vi "Capture System Configuration.vi"() -> ()   [LabVIEW 2024]
uses:
  <vilib>/Plug-In SDKs/Clients/Metadata/Test Station.ctl
  <vilib>/Plug-In SDKs/Clients/Metadata/Extension.ctl
  <vilib>/Plug-In SDKs/Clients/Metadata/Hardware Item.ctl
  <vilib>/Plug-In SDKs/Clients/Metadata/Software Item.ctl
  <vilib>/Plug-In SDKs/Clients/Metadata/Operator.ctl
  <vilib>/Plug-In SDKs/Clients/Data Store V1/Data Store Client.lvlibp/API/Data Store V1/Test Result.ctl
  <vilib>/Plug-In SDKs/Clients/Metadata/Outcome.ctl
  <vilib>/Plug-In SDKs/Clients/Metadata Store V1/Metadata Store Client.lvlibp/API/Metadata Store V1/Create Hardware Item.vi
  <vilib>/nisyscfg/Get Installed Components.vi
  <vilib>/Plug-In SDKs/Clients/Metadata Store V1/Metadata Store Client.lvlibp/API/Metadata Store V1/Create Software Item.vi
  <vilib>/Plug-In SDKs/Clients/Metadata Store V1/Metadata Store Client.lvlibp/API/Metadata Store V1/Create Test Station.vi
  <vilib>/Plug-In SDKs/Clients/Metadata Store V1/Metadata Store Client.lvlibp/API/Metadata Store V1/Create Operator.vi
  <vilib>/nisyscfg/nisyscfg.lvlib
  <resource>/objmgr/nisysapi.rc
  <vilib>/Plug-In SDKs/Clients/Metadata Store V1/Metadata Store Client.lvlibp
  <vilib>/Plug-In SDKs/Clients/Metadata/NI Metadata Types.lvlib
  <vilib>/Plug-In SDKs/Clients/Data Store V1/Data Store Client.lvlibp
panel:
  out "found operator":T1
  out "found software items":T3[](array[typedef])
  out "found hardware items":T4[](array[typedef])
  out "found test station":T5
  out "queried data":waveform(dbl)(graph)
  out "error out":errorcluster
  # "Capture System Configuration\n\nThis example uses System API to query information about the current system and create metadata items based on that information. A waveform measurement is published, then the data and metadata are read back from the published measurement."
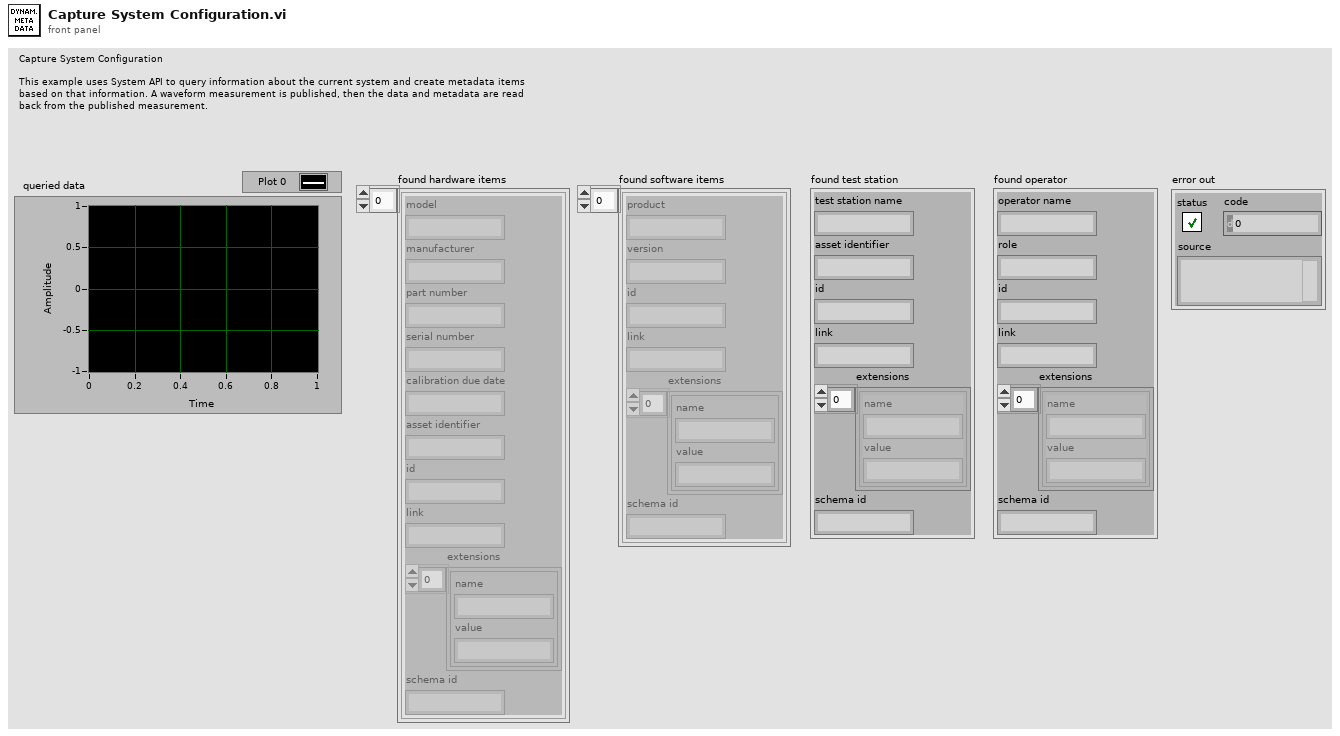
[diagram p1: front panel]
types:
  T1 = typedef "NI Metadata Types.lvlib/Operator.ctl" = cluster{"operator name":string, "role":string, "id":string, "link":string, "extensions":T2[], "schema id":string}
  T2 = typedef "NI Metadata Types.lvlib/Extension.ctl" = cluster{"name":string, "value":string}
  T3 = typedef "NI Metadata Types.lvlib/Software Item.ctl" = cluster{"product":string, "version":string, "id":string, "link":string, "extensions":T2[], "schema id":string}
  T4 = typedef "NI Metadata Types.lvlib/Hardware Item.ctl" = cluster{"model":string, "manufacturer":string, "part number":string, "serial number":string, "calibration due date":string, "asset identifier":string, "id":string, "link":string, "extensions":T2[], "schema id":string}
  T5 = typedef "NI Metadata Types.lvlib/Test Station.ctl" = cluster{"test station name":string, "asset identifier":string, "id":string, "link":string, "extensions":T2[], "schema id":string}
  T6 = typedef "Data Store Client.lvlibp/Test Result.ctl" = cluster{"test result name":string, "start date time":timestamp, "end date time":timestamp, "outcome":T7, "test result id":string, "uut instance id":string, "operator id":string, "test station id":string, "test description id":string, "software item ids":string[], "hardware item ids":string[], "test adapter ids":string[], "link":string, "extensions":T2[], "schema id":string}
  T7 = typedef "NI Metadata Types.lvlib/Outcome.ctl" = enum32{"Unspecified", "Passed", "Failed", "Indeterminate"}
  T8 = typedef "nisyscfg.lvlib/Software 1.2.ctl" = cluster{"title":string, "description":string, "ID":string, "version":string, "component type":T9}
  T9 = typedef "nisyscfg.lvlib/Component Type.ctl" = u32
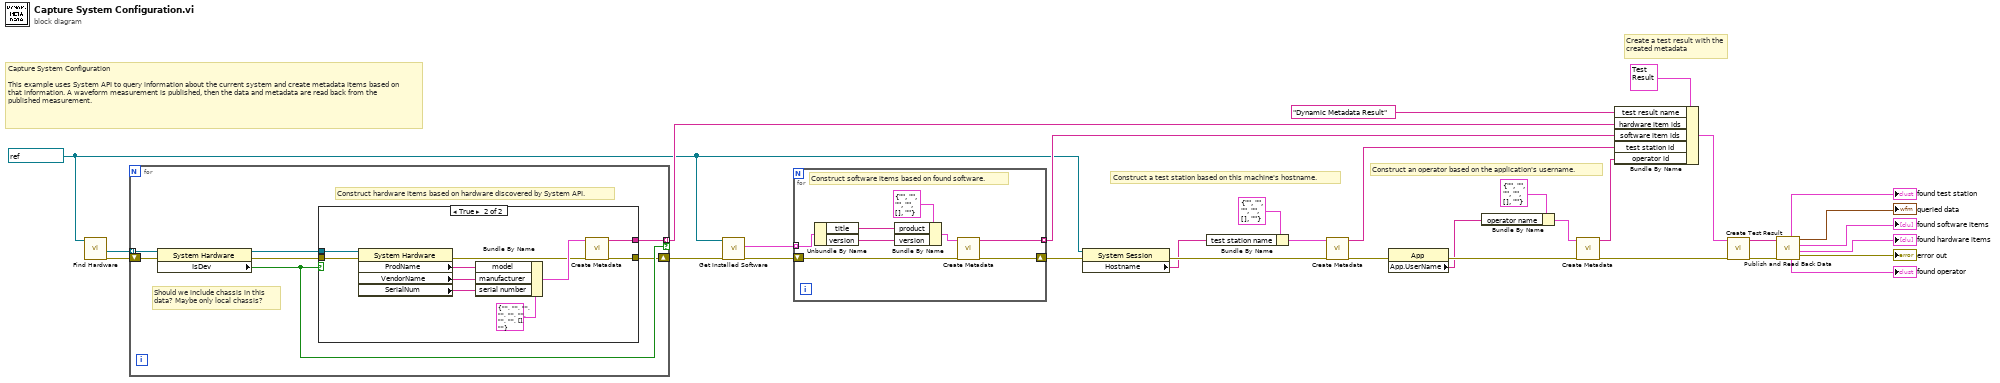
[diagram p0: block diagram]
diagram:
  w16 = refnum<k21> "localhost" ("Session in")
  # "Create a test result with the created metadata"
  # "Construct an operator based on the application's username."
  # "Capture System Configuration\n\nThis example uses System API to query information about the current system and create metadata items based on that information. A waveform measurement is published, then the data and metadata are read back from the published measurement."
  # "Construct a test station based on this machine's hostname."
  n1 = call <vilib>:"Find Hardware.vi"("Session in"=w16) -> ("error out"=w31:errorcluster, "Resources out"=w32:refnum<k20>[])  [unwired: 7 in, 2 out]
  n2 = for {
    tunnel: w32 -> [w39] mode=indexing
    tunnel: [w36] -> w17 mode=indexing if=w34
    shift-right: [w33] -> w30
    shift-left: w31 -> [w35]
    # "Construct hardware items based on hardware discovered by System API."
    # "Should we include chassis in this\ndata? Maybe only local chassis?"
    n3 = property class="System Hardware"(reference=w39, error in=w35) -> (reference out=w37:refnum<k20>, error out=w38:errorcluster, "IsDev"=w34:bool)
    n4 = case shown="True" w34 {
      tunnel: w38 -> [w40 w50]
      tunnel: w37 -> [_ w49]
      tunnel: [_ w43] -> w36
      tunnel: [w40 w41] -> w33
      frame False {
      }
      frame True {
        n5 = property class="System Hardware"(reference=w49, error in=w50) -> (error out=w42:errorcluster, "ProdName"=w46:string, "VendorName"=w45:string, "SerialNum"=w44:string)  [unwired: 1 out]
        n6 = Bundle By Name(cluster=T4 {"model"="", "manufacturer"="", "part number"="", "serial number"="", "calibration due date"="", "asset identifier"="", "id"="", "link"="", "extensions"=[], "schema id"=""} ("hardware item"), "model"=w46, "manufacturer"=w45, "serial number"=w44) -> (w48:T4)
        n7 = call-poly <vilib>:"Create Metadata.vi"("error in"=w42, "hardware item"=w48) -> ("error out"=w41:errorcluster, "hardware item id"=w43:string)  [unwired: 8 in]
      }
    }
  }
  n8 = call-poly <vilib>:"Get Installed Software.vi"("error in (no error)"=w30, "Session in"=w16) -> ("error out"=w28:errorcluster, "Software Components"=w29:T8[])  [unwired: 7 in, 1 out]
  n9 = for {
    tunnel: w29 -> [w58] mode=indexing
    shift-right: [w52] -> w25
    shift-left: w28 -> [w53]
    tunnel: [w51] -> w18 mode=indexing
    # "Construct software items based on found software."
    n10 = Unbundle By Name(w58) -> ("title"=w56:string, "version"=w55:string)
    n11 = Bundle By Name(cluster=T3 {"product"="", "version"="", "id"="", "link"="", "extensions"=[], "schema id"=""} ("software item"), "product"=w56, "version"=w55) -> (w54:T3)
    n12 = call-poly <vilib>:"Create Metadata.vi"("error in"=w53, "software item"=w54) -> ("error out"=w52:errorcluster, "software item id"=w51:string)  [unwired: 8 in]
  }
  n13 = property class="System Session"(reference=w16, error in=w25) -> (error out=w24:errorcluster, "Hostname"=w23:string)  [unwired: 1 out]
  n14 = Bundle By Name(cluster=T5 {"test station name"="", "asset identifier"="", "id"="", "link"="", "extensions"=[], "schema id"=""} ("test station"), "test station name"=w23) -> (w26:T5)
  n15 = call-poly <vilib>:"Create Metadata.vi"("error in"=w24, "test station"=w26) -> ("error out"=w6:errorcluster, "test station id"=w19:string)  [unwired: 8 in]
  n16 = property class="App"(error in=w6) -> (error out=w7:errorcluster, "App.UserName"=w3:string)  [unwired: 1 in, 1 out]
  n17 = Bundle By Name(cluster=T1 {"operator name"="", "role"="", "id"="", "link"="", "extensions"=[], "schema id"=""} ("operator metadata"), "operator name"=w3) -> (w4:T1)
  n18 = call-poly <vilib>:"Create Metadata.vi"("error in"=w7, "operator metadata"=w4) -> ("error out"=w5:errorcluster, "operator id"=w1:string)  [unwired: 8 in]
  n19 = Bundle By Name(cluster=T6 {"test result name"="", "start date time"=timestamp(0 s since 1904-01-01), "end date time"=timestamp(0 s since 1904-01-01), "outcome"=enum."Unspecified", "test result id"="", "uut instance id"="", "operator id"="", "test station id"="", "test description id"="", "software item ids"=[], "hardware item ids"=[], "test adapter ids"=[], "link"="", "extensions"=[], "schema id"=""} ("test result"), "test result name"="Dynamic Metadata Result", "hardware item ids"=w17, "software item ids"=w18, "test station id"=w19, "operator id"=w1) -> (w20:T6)
  n20 = call <vilib>:"Create Test Result.vi"("error in"=w5, "test result"=w20) -> ("error out"=w14:errorcluster, "test result id"=w15:string)  [unwired: 8 in]
  n21 = call "Publish and Read Back Data.vi"("error in (no error)"=w14, "test result id"=w15) -> ("error out"=→"error out":errorcluster, "found hardware items"=→"found hardware items":T4[], "found software items"=→"found software items":T3[], "queried data"=→"queried data":waveform(dbl), "found operator"=→"found operator":T1, "found test station"=→"found test station":T5)  [unwired: 4 in]
